vi "compress.buffer.vi"(9 "start.idx":u8, 10 "buffer.length":u8=8, 11 "buffer":u64[](array[numeric])=[4822678189205111, 0, 0, 0, 0, 0, 0, 0, 0] format="%016x") -> (2 "buffer.length.out":u8, 3 "buffer.out":u64[](array[numeric]) format="%016x")   [LabVIEW 2020]
panel:
  out "New.Val":u64 format="%016x"
  out "Even.shifted.Mask 6":u64 format="%016x"
  out "Even.shifted.Mask 5":u64 format="%016x"
  out "Even.shifted.Mask 4":u64 format="%016x"
  out "Even.Unshifted.Mask 3":u64 format="%016x"
  out "Remainder.len":u8
  out "Even.Result 2":u64 format="%016x"
  out "Even.Unshifted.Mask 2":u64 format="%016x"
  out "Even.Result":u64 format="%016x"
  out "Even.Mask":u64 format="%016x"
  out "Even.Unshifted.Mask":u64 format="%.0x"
  out "Word":u8
  out "Remainder.idx":u8
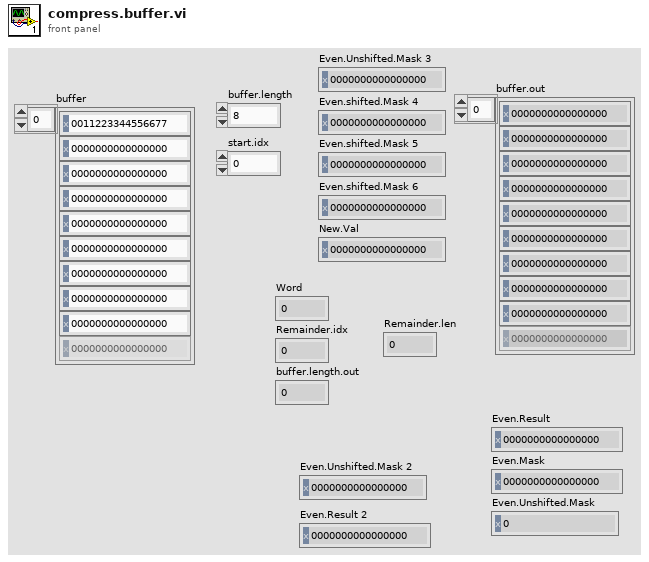
[diagram p1: front panel]
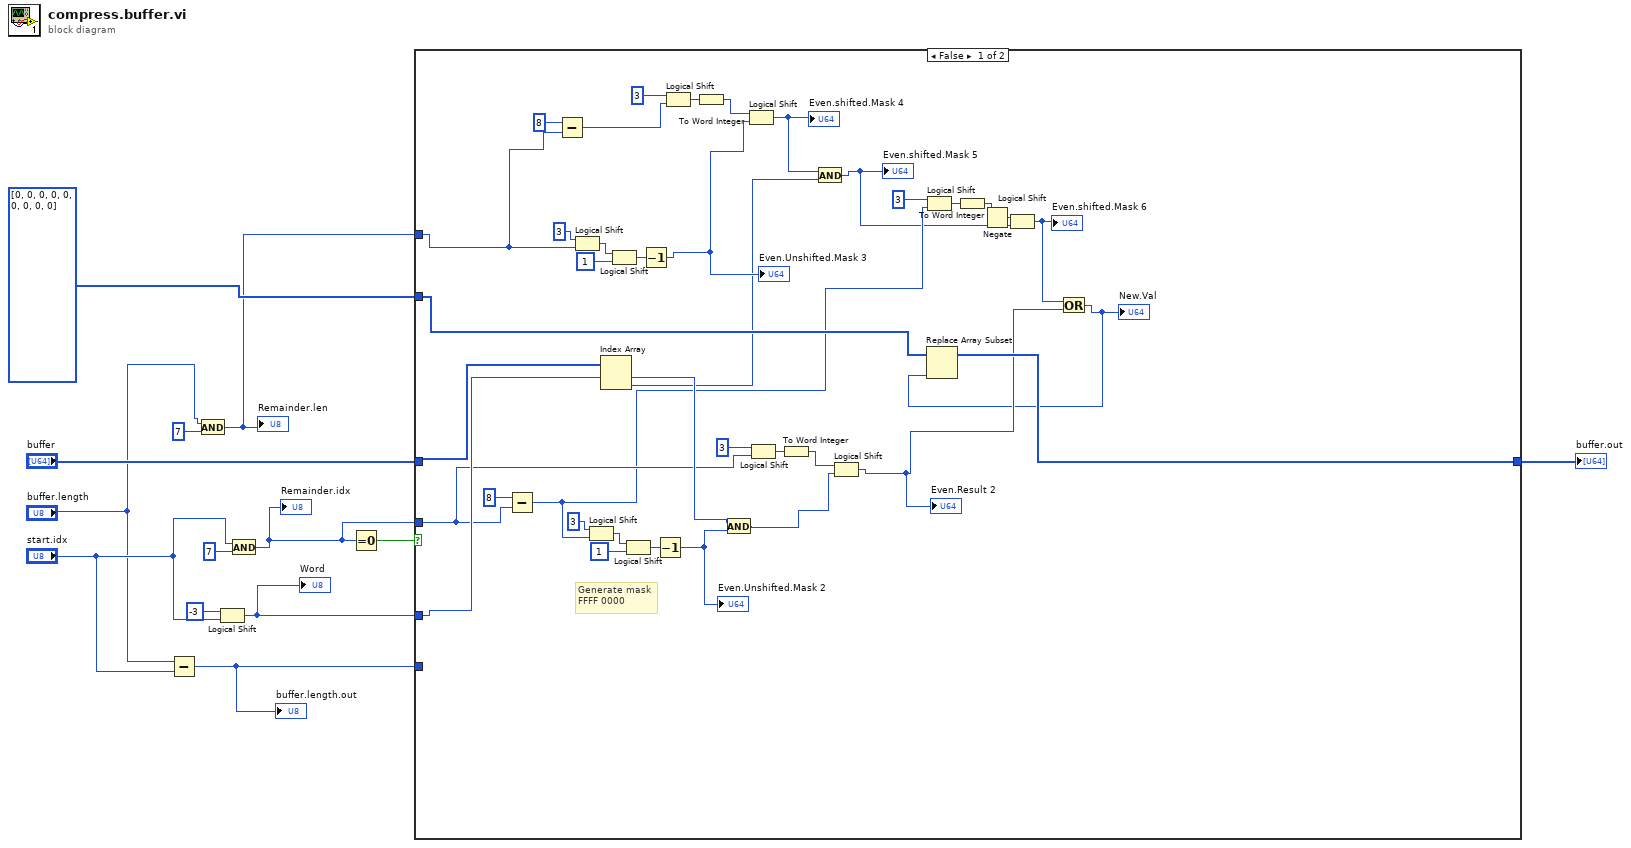
[diagram p0: block diagram]
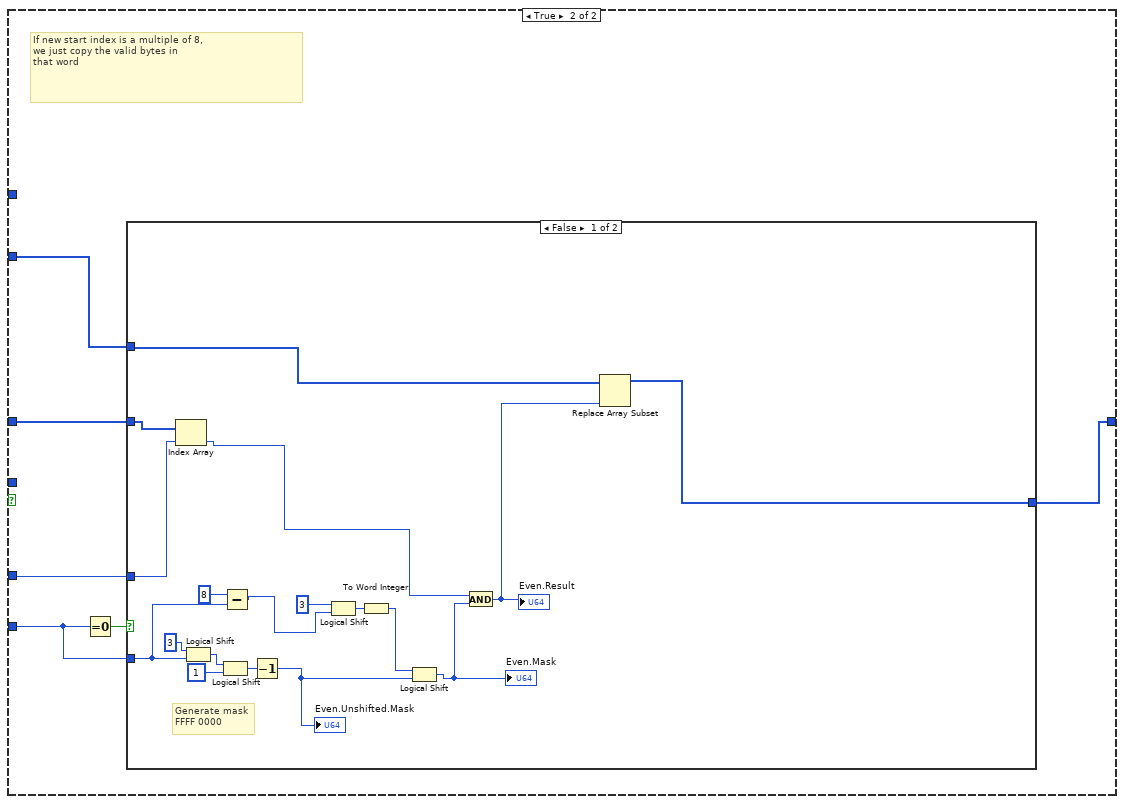
[diagram p2: hidden frame]
diagram:
  n1 = Subtract(x="buffer.length", y="start.idx") -> (x-y=w6:u8)
  "buffer.length.out" <- w6
  n2 = And(x="buffer.length", y=u8 7) -> (x .and. y?=w1:u8)
  "Remainder.len" <- w1
  n3 = Logical Shift(y=i16 -3, x="start.idx") -> (x << y=w9:u8)
  "Word" <- w9
  n4 = And(x="start.idx", y=u8 7) -> (x .and. y?=w4:u8)
  "Remainder.idx" <- w4
  n5 = Equal To 0?(x=w4) -> (x = 0?=w11:bool)
  n6 = case shown="False" w11 {
    tunnel: "buffer" -> [w46 w57]
    tunnel: w9 -> [w45 w54]
    tunnel: [w36 w55] -> w8
    tunnel: w6 -> [_ w53]
    tunnel: u64[] [0, 0, 0, 0, 0, 0, 0, 0, 0] ("buffer.out 2") -> [w37 w52]
    tunnel: w4 -> [w38 _]
    tunnel: w1 -> [w28 _]
    frame False {
      # "Generate mask\nFFFF 0000"
      n7 = Subtract(x=u8 8, y=w38) -> (x-y=w19:u8)
      n8 = Subtract(x=u8 8, y=w28) -> (x-y=w27:u8)
      n9 = Logical Shift(y=i16 3, x=w28) -> (x << y=w32:u8)
      n10 = Logical Shift(y=i16 3, x=w19) -> (x << y=w48:u8)
      n11 = Index Array(array=w46, index #1=w45) -> (element #1=w43:u64, element #2=w23:u64)  [unwired: 1 in]
      n12 = Logical Shift(y=w32, x=u64 1) -> (x << y=w34:u64)
      n13 = Logical Shift(y=w48, x=u64 1) -> (x << y=w50:u64)
      n14 = Decrement(x=w34) -> (x-1=w24:u64)
      "Even.Unshifted.Mask 3" <- w24
      n15 = Decrement(x=w50) -> (x-1=w44:u64)
      "Even.Unshifted.Mask 2" <- w44
      n16 = Logical Shift(y=i16 3, x=w27) -> (x << y=w30:u8)
      n17 = To Word Integer(number=w30) -> (16bit integer=w29:i16)
      n18 = And(x=w43, y=w44) -> (x .and. y?=w40:u64)
      n19 = Logical Shift(y=w29, x=w24) -> (x << y=w25:u64)
      "Even.shifted.Mask 4" <- w25
      n20 = Logical Shift(y=i16 3, x=w38) -> (x << y=w41:u8)
      n21 = To Word Integer(number=w41) -> (16bit integer=w39:i16)
      n22 = And(x=w25, y=w23) -> (x .and. y?=w18:u64)
      "Even.shifted.Mask 5" <- w18
      n23 = Logical Shift(y=w39, x=w40) -> (x << y=w15:u64)
      "Even.Result 2" <- w15
      n24 = Logical Shift(y=i16 3, x=w19) -> (x << y=w21:u8)
      n25 = To Word Integer(number=w21) -> (16bit integer=w20:i16)
      n26 = Negate(x=w20) -> (-x=w17:i16)
      n27 = Logical Shift(y=w17, x=w18) -> (x << y=w16:u64)
      "Even.shifted.Mask 6" <- w16
      n28 = Or(x=w16, y=w15) -> (x .or. y?=w14:u64)
      "New.Val" <- w14
      n29 = Replace Array Subset(array=w37, new element=w14) -> (w36:u64[])  [unwired: 1 in]
    }
    frame True {
      # "If new start index is a multiple of 8,\nwe just copy the valid bytes in \nthat word"
      n30 = Equal To 0?(x=w53) -> (x = 0?=w56:bool)
      n31 = case shown="False" w56 {
        tunnel: w57 -> [w73 _]
        tunnel: [w74 w76] -> w55
        tunnel: w52 -> [w75 w76]
        tunnel: w54 -> [w72 _]
        tunnel: w53 -> [w65 _]
        frame False {
          # "Generate mask\nFFFF 0000"
          n32 = Index Array(array=w73, index=w72) -> (element=w60:u64)
          n33 = Logical Shift(y=i16 3, x=w65) -> (x << y=w68:u8)
          n34 = Logical Shift(y=w68, x=u64 1) -> (x << y=w70:u64)
          n35 = Subtract(x=u8 8, y=w65) -> (x-y=w63:u8)
          n36 = Decrement(x=w70) -> (x-1=w61:u64)
          "Even.Unshifted.Mask" <- w61
          n37 = Logical Shift(y=i16 3, x=w63) -> (x << y=w66:u8)
          n38 = To Word Integer(number=w66) -> (16bit integer=w62:i16)
          n39 = Logical Shift(y=w62, x=w61) -> (x << y=w59:u64)
          "Even.Mask" <- w59
          n40 = And(x=w60, y=w59) -> (x .and. y?=w58:u64)
          "Even.Result" <- w58
          n41 = Replace Array Subset(array=w75, new element=w58) -> (w74:u64[])  [unwired: 1 in]
        }
        frame True {
        }
      }
    }
  }
  "buffer.out" <- w8
